vi "Compute Decay & Time Gates.vi"(6 "Version":enum32{"Version 1", "Version 2"}(radio), 8 "Error In":errorcluster, 9 "Decay & Gates Options":T3, 10 "Gates Definitions":T6={"First Gate: t1"=0.0, "Gate Width: W"=4.0, "Gate Step: d"=0.3, "# Gates: G"=50.0, "Use Gate Center"=FALSE, "Frames/Image: F"=50, "Gates/Frame: L"=0, "Bits/Frame: q"=0, "Multiplicity: p"=0, "Gate Type"=enum."Square", "Gate Edge s"=4.0, "Gate Top Slope"=4.0, "Reversed Sawtooth?"=FALSE, "Computation"=FALSE, "User-defined Gate"={"X Array"=[], "Y Array"=[]}, "Tolerance"=50.0, "Integration"=enum."Item 0", "# Steps"=50.0, "Type of User-defined Function"=enum."Gate"}, 11 "Decay Definition":T4={"offset: t0"=2.0, "period: T"=15.0, "lifetime: tau"=0.5, "Incident Signal: I"=0.5, "Normalized Decays"=FALSE, "IRF Model"=enum."Dirac", "IRF Parameter 1"=0.0}) -> (0 "Error Out":errorcluster, 1 "Gate Sum":dbl, 2 "Plot Names":string[](array[string]), 3 "Plots":cluster{"t Array":dbl[], "Gate Array":dbl[]}[](array[cluster]), 4 "Decay Analysis Results":T1 {"A" format="%#_5g"; "tau" format="%#_5g"; "Bkgd" format="%#_5g"; "Min" format="%#_5g"; "Max" format="%#_5g"}, 5 "Scales":cluster{"X Scale":u32, "Y Scale":u32}[](array[cluster]), 7 "Plots Interpolation (Previous Plot's Style)":T2[](array[typedef]) items=["Point (.)", "Stepwise Right (--.)", "Line + Point (\\. /)", "Stepwise Left (.--)", "Stepwise Centered (-.-)", "Stepwise Vertical (|.|)", "Line (-)", "Use Previous Plot's Style"])   [LabVIEW 2019]
uses:
  Gate Definitions.ctl
  Gate Type.ctl
  XY Plot Data.ctl
  Decay Definiton.ctl
  IRF Model.ctl
  Decay & Gates Options.ctl
  LabVIEW Plot Interpolation.ctl
  Gate Analysis Results.ctl
  Linear Ramp End Options.ctl
  8f995b8f-6563-4a36-b24f-17447402644a.vi/69b89faf-335b-4e54-b1eb-c494efef2307.vi
  Square Gated 1-Exp Parameters.ctl
  <vilib>/gmath/NI_Gmath.lvlib
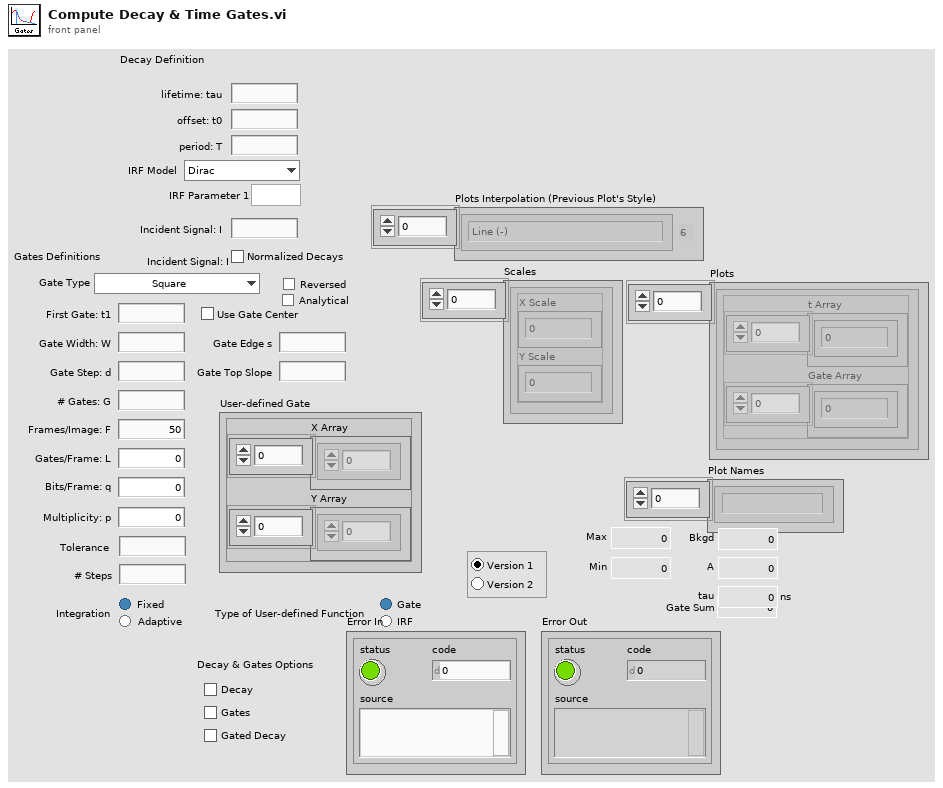
[diagram p1: front panel]
types:
  T1 = typedef "Gate Analysis Results.ctl" = cluster{"Max":dbl, "Min":dbl, "Bkgd":dbl, "tau ":dbl[unit], "A":dbl}
  T2 = typedef "LabVIEW Plot Interpolation.ctl" = u8
  T3 = typedef "Decay & Gates Options.ctl" = cluster{"Decay":bool, "Gate":bool, "Gated Decay":bool}
  T4 = typedef "Decay Definiton.ctl" = cluster{"offset: t0":ext, "period: T":ext, "lifetime: tau":ext, "Incident Signal: I":ext, "Normalized Decays":bool, "IRF Model":T5, "IRF Parameter 1":ext}
  T5 = typedef "IRF Model.ctl" = enum16{"Dirac", "Exponential"}
  T6 = typedef "Gate Definitions.ctl" = cluster{"First Gate: t1":ext, "Gate Width: W":ext, "Gate Step: d":ext, "# Gates: G":ext, "Use Gate Center":bool, "Frames/Image: F":i32, "Gates/Frame: L":i32, "Bits/Frame: q":i32, "Multiplicity: p":i32, "Gate Type":T7, "Gate Edge s":ext, "Gate Top Slope":ext, "Reversed Sawtooth?":bool, "Computation":bool, "User-defined Gate":T8, "Tolerance":ext, "Integration":enum32{"Item 0", "Item 1"}, "# Steps":ext, "Type of User-defined Function":enum32{"Gate", "IRF"}}
  T7 = typedef "Gate Type.ctl" = enum16{"Square", "Finite Edge Square", "Finite Edge, Tilted Top Square", "Triangle", "Sawtooth", "User-defined"}
  T8 = typedef "XY Plot Data.ctl" = cluster{"X Array":dbl[], "Y Array":dbl[]}
  T9 = typedef "Linear Ramp End Options.ctl" = enum16{"Include Min/Exclude Max", "Exclude Min/Include Max", "Include Both Ends", "Exclude Both Ends"}
  T10 = typedef "Square Gated 1-Exp Parameters.ctl" = cluster{"P-R":dbl, "W":dbl, "T":dbl}
  T11 = cluster{"t Array":ext[], "Gate Image Array":ext[]}
  T12 = cluster{"t Array":ext[], "Gate Image Array":ext[]}[]
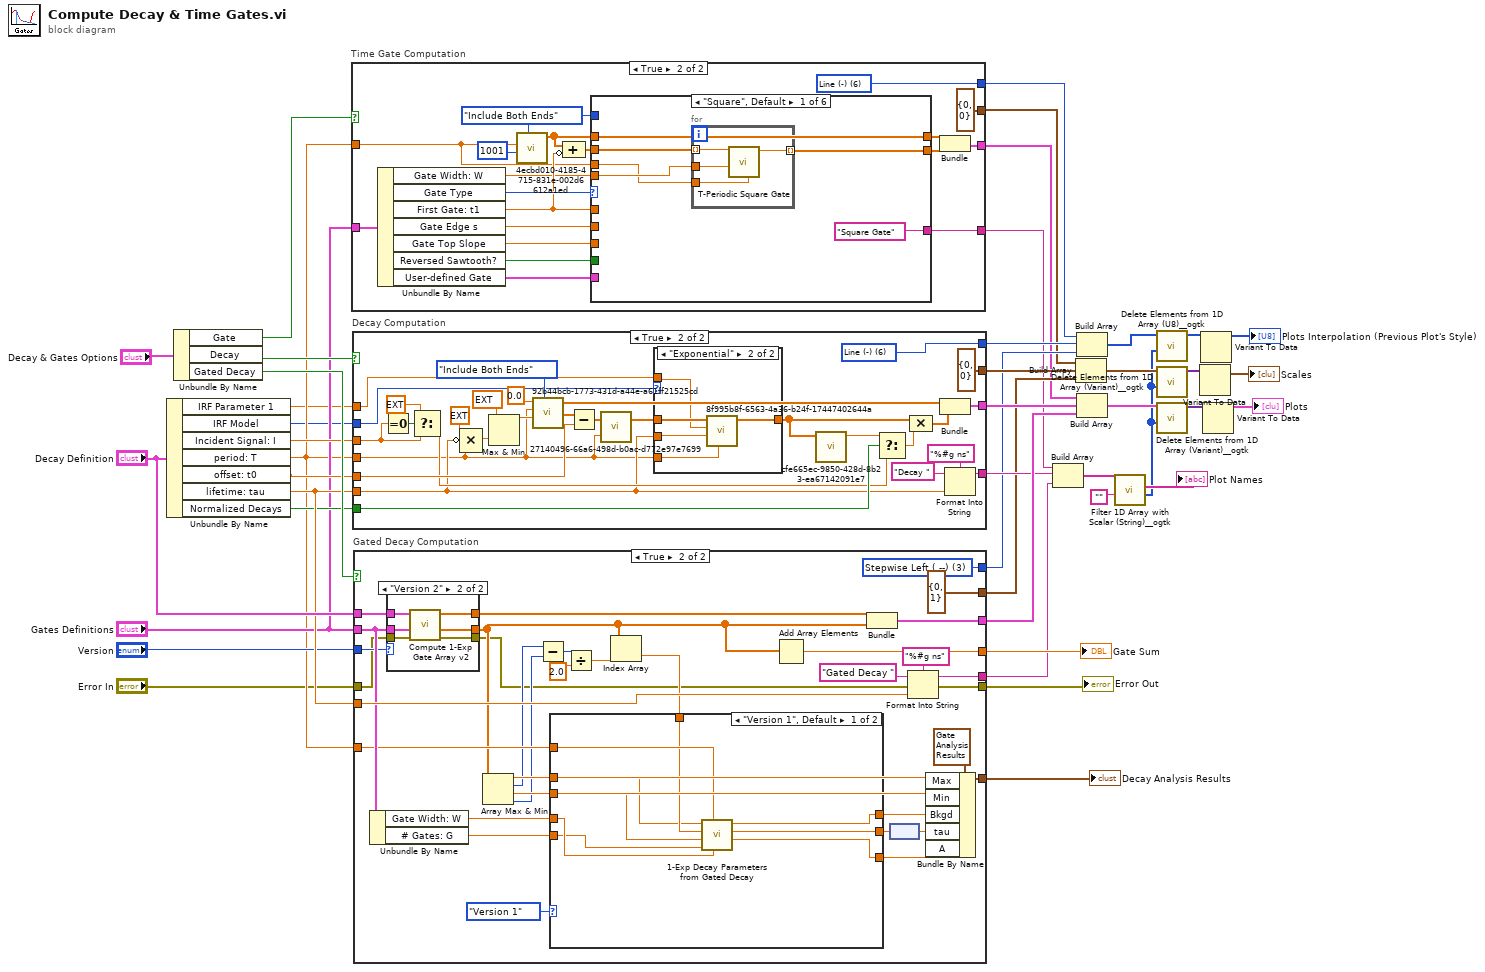
[diagram p0: block diagram]
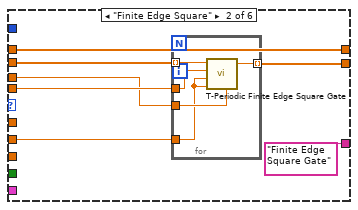
[diagram p3: hidden frame]
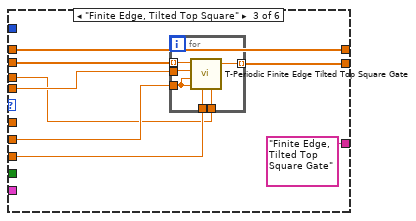
[diagram p4: hidden frame]
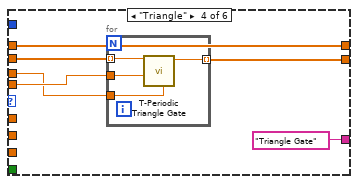
[diagram p5: hidden frame]
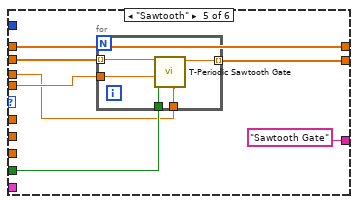
[diagram p6: hidden frame]
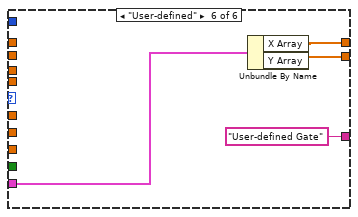
[diagram p7: hidden frame]
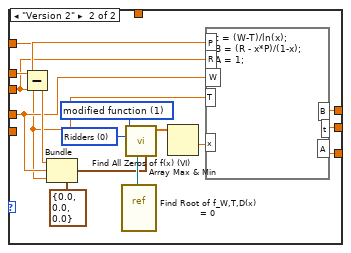
[diagram p9: hidden frame]
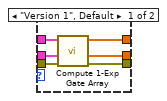
[diagram p10: hidden frame]
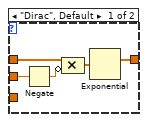
[diagram p12: hidden frame]
diagram:
  n1 = Unbundle By Name("Decay Definition") -> ("IRF Parameter 1"=w3:ext, "IRF Model"=w4:T5, "Incident Signal: I"=w13:ext, "period: T"=w5:ext, "offset: t0"=w16:ext, "lifetime: tau"=w35:ext, "Normalized Decays"=w11:bool)
  n2 = Unbundle By Name("Decay & Gates Options") -> ("Gate"=w12:bool, "Decay"=w39:bool, "Gated Decay"=w38:bool)
  n3 = case "Time Gate Computation" shown="True" w12 {
    tunnel: [_ w62] -> w7
    tunnel: [_ cluster{"X Scale":u32, "Y Scale":u32} {"X Scale"=0, "Y Scale"=0} ("Cluster")] -> w8
    tunnel: [_ w60] -> w9
    tunnel: "Gates Definitions" -> [_ w59]
    tunnel: [_ w56] -> w6
    tunnel: w5 -> [_ w44]
    frame False {
    }
    frame True {
      w60 = T2 6 items=["Point (.)", "Stepwise Right (--.)", "Line + Point (\\. /)", "Stepwise Left (.--)", "Stepwise Centered (-.-)", "Stepwise Vertical (|.|)", "Line (-)", "Use Previous Plot's Style"] ("Plots Interpolation (Previous Plot's Style)")
      w51 = Linear_Ramp_End_Options."Include Both Ends" ("Options")
      n4 = Unbundle By Name(w59) -> ("Gate Width: W"=w50:ext, "Gate Type"=w58:T7, "First Gate: t1"=w55:ext, "Gate Edge s"=w54:ext, "Gate Top Slope"=w53:ext, "Reversed Sawtooth?"=w46:bool, "User-defined Gate"=w45:T8)
      n5 = call "4ecbd010-4185-4715-831e-002d6612a1ed.vi"("Options"=w51, "# Steps (1)"=1001 ("# Steps"), "End (1)"=w44) -> ("Ramp"=w48:ext[])  [unwired: 7 in, 1 out]
      n6 = Compound Arithmetic op=ADD(w48, invert w55) -> (w49:ext[])
      n7 = case shown="\"Square\", Default" w58 {
        tunnel: w49 -> [w67 w75 w87 w103 w114 _]
        tunnel: w55 -> [_ _ _ _ _ _]
        tunnel: [w65 w78 w91 w101 w112 w123] -> w57
        tunnel: ["Square Gate" "Finite Edge Square Gate" "Finite Edge, Tilted Top Square Gate" "Triangle Gate" "Sawtooth Gate" "User-defined Gate"] -> w56
        tunnel: w50 -> [w66 w76 w89 w102 w113 _]
        tunnel: w54 -> [_ w77 w88 _ _ _]
        tunnel: w53 -> [_ _ w90 _ _ _]
        tunnel: w51 -> [_ _ _ _ _ _]
        tunnel: w48 -> [w64 w74 w86 w100 w111 _]
        tunnel: [w64 w74 w86 w100 w111 w122] -> w47
        tunnel: w46 -> [_ _ _ _ w110 _]
        tunnel: w45 -> [_ _ _ _ _ w121]
        tunnel: w44 -> [w63 w73 w85 w99 w109 _]
        frame "Square", Default {
          n8 = for {
            tunnel: w67 -> [w72] mode=indexing
            tunnel: w66 -> [w71]
            tunnel: [w70] -> w65 mode=indexing
            tunnel: w63 -> [w69]
            n9 = call "T-Periodic Square Gate.vi"("Period T"=w69, "W"=w71, "t"=w72) -> ("Square(t)"=w70:dbl)  [unwired: 8 in]
          }
        }
        frame "Finite Edge Square" {
          n10 = for {
            tunnel: [w84] -> w78 mode=indexing
            tunnel: w76 -> [w83]
            tunnel: w77 -> [w80]
            tunnel: w75 -> [w82] mode=indexing
            tunnel: w73 -> [w81]
            n11 = call "T-Periodic Finite Edge Square Gate.vi"("Period T"=w81, "s_F"=w80, "s_R"=w80, "W"=w83, "t"=w82) -> ("Finite Edge Square(t)"=w84:dbl)  [unwired: 6 in]
          }
        }
        frame "Finite Edge, Tilted Top Square" {
          n12 = for {
            tunnel: [w98] -> w91 mode=indexing
            tunnel: w89 -> [w97]
            tunnel: w88 -> [w95]
            tunnel: w90 -> [w94]
            tunnel: w87 -> [w96] mode=indexing
            tunnel: w85 -> [w93]
            n13 = call "T-Periodic Finite Edge Tilted Top Square Gate.vi"("Period T"=w93, "slope"=w94, "s_F"=w95, "s_R"=w95, "W"=w97, "t"=w96) -> ("Finite Edge Square(t)"=w98:dbl)  [unwired: 5 in]
          }
        }
        frame "Triangle" {
          n14 = for {
            tunnel: w103 -> [w108] mode=indexing
            tunnel: w102 -> [w107]
            tunnel: [w106] -> w101 mode=indexing
            tunnel: w99 -> [w105]
            n15 = call "T-Periodic Triangle Gate.vi"("Period T"=w105, "W"=w107, "t"=w108) -> ("Triangle(t)"=w106:dbl)  [unwired: 8 in]
          }
        }
        frame "Sawtooth" {
          n16 = for {
            tunnel: w114 -> [w120] mode=indexing
            tunnel: w113 -> [w119]
            tunnel: [w118] -> w112 mode=indexing
            tunnel: w110 -> [w117]
            tunnel: w109 -> [w116]
            n17 = call "T-Periodic Sawtooth Gate.vi"("Period T"=w116, "Reversed?"=w117, "W"=w119, "t"=w120) -> ("Sawtooth(t)"=w118:dbl)  [unwired: 7 in]
          }
        }
        frame "User-defined" {
          n18 = Unbundle By Name(w121) -> ("X Array"=w122:dbl[], "Y Array"=w123:dbl[])
        }
      }
      n19 = Bundle("Ramp"=w47, "Y Array"=w57) -> (w62:cluster{"Ramp":ext[], "Y Array":dbl[]})  [unwired: 1 in]
    }
  }
  n20 = case "Decay Computation" shown="True" w39 {
    tunnel: [_ w151] -> w43
    tunnel: [_ w145] -> w37
    tunnel: w35 -> [_ w133]
    tunnel: [_ cluster{"X Scale":u32, "Y Scale":u32} {"X Scale"=0, "Y Scale"=0} ("Cluster")] -> w27
    tunnel: [_ w143] -> w22
    tunnel: w5 -> [_ w126]
    tunnel: w16 -> [_ w142]
    tunnel: w13 -> [_ w139]
    tunnel: w11 -> [_ w138]
    tunnel: w4 -> [_ w128]
    tunnel: w3 -> [_ w127]
    frame False {
    }
    frame True {
      w143 = T2 6 items=["Point (.)", "Stepwise Right (--.)", "Line + Point (\\. /)", "Stepwise Left (.--)", "Stepwise Centered (-.-)", "Stepwise Vertical (|.|)", "Line (-)", "Use Previous Plot's Style"] ("Plots Interpolation (Previous Plot's Style)")
      n21 = Equal To 0?(x=w139) -> (x = 0?=w141:bool)
      n22 = Select(t=ext 1.0, s=w141, f=w139) -> (s? t:f=w136:ext)
      n23 = Compound Arithmetic op=MULTIPLY(ext 10.0 ("value"), invert w133, w126) -> (w131:ext)
      n24 = Max & Min(x=ext 1001.0, y=w131) -> (max(x,y)=w129:ext)  [unwired: 1 out]
      n25 = call "92b44bcb-1773-431d-a44e-a61ff21525cd.vi"("Options"=Linear_Ramp_End_Options."Include Both Ends", "# Steps (1)"=w129, "End (1)"=w126, "Start (0)"=0.0 ("Min")) -> ("Ramp"=w152:ext[])  [unwired: 6 in, 1 out]
      n26 = Subtract(x=w152, y=w142) -> (x-y=w149:ext[])
      n27 = call "27140496-66a6-498d-b0ac-d772e97e7699.vi"("y"=w126, "x"=w149) -> ("x - E(x/y)y"=w148:ext[])  [unwired: 1 out]
      n28 = case shown="\"Exponential\"" w128 {
        tunnel: w148 -> [w158 w163]
        tunnel: [w155 w159] -> w125
        tunnel: w133 -> [w154 w161]
        tunnel: w127 -> [_ w162]
        tunnel: w126 -> [_ w160]
        frame "Dirac", Default {
          n29 = Negate(x=w154) -> (-x=w157:ext)
          n30 = Compound Arithmetic op=MULTIPLY(w158, invert w157) -> (w156:ext[])
          n31 = Exponential(1:w156) -> (0:w155:ext[])
        }
        frame "Exponential" {
          n32 = call "8f995b8f-6563-4a36-b24f-17447402644a.vi"("Period: T"=w160, "lifetime: tau"=w161, "IRF time constant"=w162, "t"=w163) -> ("y(t)"=w159:ext[])  [unwired: 6 in, 1 out]
        }
      }
      n33 = call "cfe665ec-9850-428d-8b23-ea67142091e7.vi"("y(t)"=w125) -> ("Peak Normalization Factor"=w134:ext)  [unwired: 10 in]
      n34 = Select(t=w134, s=w138, f=w136) -> (s? t:f=w135:ext)
      n35 = Compound Arithmetic op=MULTIPLY(w125, w135) -> (w137:ext[])
      n36 = Bundle("Ramp"=w152, w137) -> (w151:cluster{"Ramp":ext[], ext[]})  [unwired: 1 in]
      n37 = Format Into String(format string="%#g ns", initial string="Decay ", w133) -> (resulting string=w145:string)  [unwired: 1 in, 1 out]
    }
  }
  n38 = case "Gated Decay Computation" shown="True" w38 {
    tunnel: [_ w198] -> w42
    tunnel: "Decay Definition" -> [_ w197]
    tunnel: "Gates Definitions" -> [_ w190]
    tunnel: [_ w196] -> w41
    tunnel: w35 -> [_ w194]
    tunnel: [_ w193] -> w34
    tunnel: [_ cluster{"X Scale":u32, "Y Scale":i32} {"X Scale"=0, "Y Scale"=1} ("Cluster")] -> w26
    tunnel: [_ w191] -> w21
    tunnel: w5 -> [_ w181]
    tunnel: [_ w188] -> w15
    tunnel: "Version" -> [_ w172]
    tunnel: "Error In" -> [w164 w167]
    tunnel: [w164 w165] -> w1
    frame False {
    }
    frame True {
      w191 = T2 3 items=["Point (.)", "Stepwise Right (--.)", "Line + Point (\\. /)", "Stepwise Left (.--)", "Stepwise Centered (-.-)", "Stepwise Vertical (|.|)", "Line (-)", "Use Previous Plot's Style"] ("Plots Interpolation (Previous Plot's Style)")
      n39 = Unbundle By Name(w190) -> ("Gate Width: W"=w182:ext, "# Gates: G"=w168:ext)
      n40 = case shown="\"Version 2\"" w172 {
        tunnel: w197 -> [w228 w234]
        tunnel: w190 -> [w227 w233]
        tunnel: [w226 w232] -> w179
        tunnel: [w225 w231] -> w174
        tunnel: [w223 w230] -> w166
        tunnel: w167 -> [w224 w229]
        frame "Version 1", Default {
          n41 = call "Compute 1-Exp Gate Array.vi"("Error In"=w224, "Gates Definitions"=w227, "Decay Definition"=w228) -> ("Error Out"=w223:errorcluster, "Gate Array"=w225:dbl[], "t Array"=w226:dbl[])  [unwired: 6 in]
        }
        frame "Version 2" {
          n42 = call "Compute 1-Exp Gate Array v2.vi"("Error In"=w229, "Gates Definitions"=w233, "Decay Definition"=w234) -> ("Error Out"=w230:errorcluster, "Gate Image Array"=w231:ext[], "t Array"=w232:ext[])  [unwired: 4 in, 2 out]
        }
      }
      n43 = Array Max & Min(array=w174) -> (max value=w187:ext, max index (indices)=w178:i32, min value=w186:ext, min index (indices)=w177:i32)
      n44 = Subtract(x=w178, y=w177) -> (x-y=w176:i32)
      n45 = Divide(x=w176, y=2.0) -> (x/y=w175:dbl)
      n46 = Index Array(array=w174, index=w175) -> (element=w173:ext)
      n47 = case shown="\"Version 1\", Default" enum32{"Version 1", "Version 2"}."Version 1" ("Version") {
        tunnel: w187 -> [w200 w215]
        tunnel: w186 -> [w202 w214]
        tunnel: [w207 w216] -> w185
        tunnel: [w206 w213] -> w184
        tunnel: w182 -> [w205 w212]
        tunnel: w181 -> [w204 w211]
        tunnel: w173 -> [w201 _]
        tunnel: [w203 w208] -> w169
        tunnel: w168 -> [w199 _]
        frame "Version 1", Default {
          n48 = call "1-Exp Decay Parameters from Gated Decay.vi"("Gate Width: W"=w205, "period: T"=w204, "# Gates"=w199, "Min Decay"=w202, "Mid Decay"=w201, "Max Decay"=w200) -> ("x"=w203:dbl, "tau"=w206:dbl, "B"=w207:dbl)  [unwired: 2 in, 1 out]
        }
        frame "Version 2" {
          w221 = u16 0 items=["Ridders", "Newton Raphson"] ("algorithm")
          w222 = u16 1 items=["fixed function", "modified function"] ("step type")
          n49 = Subtract(x=w215, y=w214) -> (x-y=w220:ext)
          n50 = Bundle(cluster=T10 {"P-R"=0.0, "W"=0.0, "T"=0.0} ("Square Gated Single Exponential Parameters"), "P-R"=w220, "W"=w212, "T"=w211) -> (w218:T10)
          n51 = vi-ref "Find Root of f_W,T,D(x) = 0.vi"() -> (w219:refnum<vi>)
          n52 = call <vilib>:"Find All Zeros of f(x) (VI).vi"("data"=w218, "f(x)"=w219, "algorithm"=w221, "step type"=w222) -> ("Zeros"=w217:dbl[])  [unwired: 4 in, 3 out]
          n53 = Array Max & Min(array=w217) -> (min value=w210:dbl)  [unwired: 3 out]
          n54 = formula code="t = (W-T)/ln(x);\nB = (R - x*P)/(1-x);\nA = 1;"("P"=w215, "R"=w214, "x"=w210, "W"=w212, "T"=w211) -> ("B"=w216:dbl, "t"=w213:dbl, "A"=w208:dbl)
        }
      }
      n55 = Add Array Elements(numeric array=w174) -> (sum=w196:ext)
      n56 = Bundle("t Array"=w179, "Gate Image Array"=w174) -> (w198:T11)  [unwired: 1 in]
      n57 = node(w184) -> (w183:dbl[unit])
      n58 = Format Into String(format string="%#g ns", initial string="Gated Decay ", error in=w166, w194) -> (resulting string=w193:string, error out=w165:errorcluster)
      n59 = Bundle By Name(cluster=T1 {"Max"=19.0, "Min"=19.0, "Bkgd"=19.0, "tau "=1.9e-08, "A"=0.0} ("Decay Analysis Results"), "Max"=w187, "Min"=w186, "Bkgd"=w185, "tau"=w183, "A"=w169) -> (w188:T1)
    }
  }
  "Gate Sum" <- w41
  "Error Out" <- w1
  "Decay Analysis Results" <- w15
  n60 = Build Array(w6, w37, w34) -> (w33:string[])
  n61 = Build Array(w8, w27, w26) -> (w25:cluster{"X Scale":u32, "Y Scale":u32}[])
  n62 = Build Array(w9, w22, w21) -> (w20:T2[])
  n63 = Build Array(w7, w43, w42) -> (w30:T12)
  n64 = call <userlib>:"Filter 1D Array with Scalar (String)__ogtk.vi"("items to filter"="", "array"=w33) -> ("filtered item indices"=w19:i32[], "filtered array"=→"Plot Names":string[])  [unwired: 4 in]
  n65 = call <userlib>:"Delete Elements from 1D Array (U8)__ogtk.vi"("indices"=w19, "array"=w20) -> ("array w/ subset deleted"=w18:u8[])  [unwired: 8 in, 1 out]
  n66 = call <userlib>:"Delete Elements from 1D Array (Variant)__ogtk.vi"("indices"=w19, "array"=w25) -> ("array w/ subset deleted"=w24:variant[])  [unwired: 8 in, 1 out]
  n67 = call <userlib>:"Delete Elements from 1D Array (Variant)__ogtk.vi"("indices"=w19, "array"=w30) -> ("array w/ subset deleted"=w29:variant[])  [unwired: 8 in, 1 out]
  n68 = Variant To Data(Variant=w24) -> (data=→"Scales":cluster{"X Scale":u32, "Y Scale":u32}[])  [unwired: 2 in, 1 out]
  n69 = Variant To Data(Variant=w18) -> (data=→"Plots Interpolation (Previous Plot's Style)":T2[])  [unwired: 2 in, 1 out]
  n70 = Variant To Data(Variant=w29) -> (data=→"Plots":cluster{"t Array":dbl[], "Gate Array":dbl[]}[])  [unwired: 2 in, 1 out]
